vi "Parent Interfaces.vi"(8 "error in":errorcluster, 10 "Path":path) -> (0 "error out":errorcluster, 2 "Parent Interface Paths":path[](array[path]))   [LabVIEW 2020, in "jettl.lvlib" / "Actor.lvlib"]
uses:
  Actor.lvlib
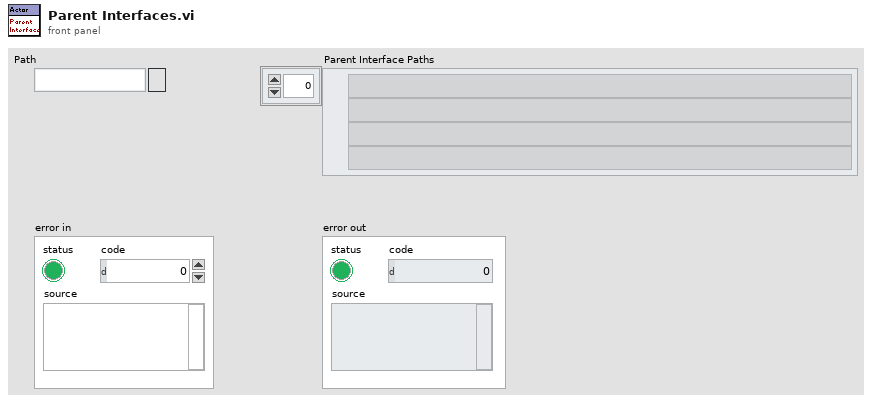
[diagram p1: front panel]
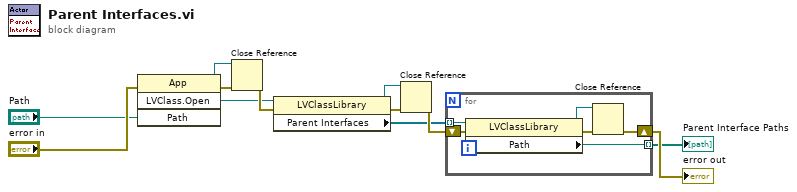
[diagram p0: block diagram]
diagram:
  n1 = invoke class="App" method="LVClass.Open"(error in="error in", "Path"="Path") -> (reference out=w12:refnum<vi>, error out=w11:errorcluster, "LVClass.Open"=w9:refnum<vi>)  [unwired: 2 in, 1 out]
  n2 = Close Reference(reference=w12, error in (no error)=w11) -> (error out=w10:errorcluster)
  n3 = property class="LVClassLibrary"(reference=w9, error in=w10) -> (reference out=w7:refnum<vi>, error out=w8:errorcluster, "Parent Interfaces"=w5:refnum<vi>[])
  n4 = Close Reference(reference=w7, error in (no error)=w8) -> (error out=w6:errorcluster)
  n5 = for {
    tunnel: w5 -> [w17] mode=indexing
    shift-right: [w14] -> w4
    shift-left: w6 -> [w18]
    tunnel: [w13] -> w3 mode=indexing
    n6 = property class="LVClassLibrary"(reference=w17, error in=w18) -> (reference out=w15:refnum<vi>, error out=w16:errorcluster, "Path"=w13:path)
    n7 = Close Reference(reference=w15, error in (no error)=w16) -> (error out=w14:errorcluster)
  }
  "error out" <- w4
  "Parent Interface Paths" <- w3
